vi "Set Level.vi"(6 "Output Channel":T1, 8 "error in (no error)":errorcluster, 9 "Slew (V/s)":dbl, 10 "Level (V)":dbl, 11 "RP100 in":refnum<class "RP100.lvclass">) -> (0 "error out":errorcluster, 3 "RP100 out":refnum<class "RP100.lvclass">)   [LabVIEW 2019, in "RP100.lvclass"]
doc: "Set the output <b>Level</b> with <b>Slew</b> rate on the selected <b>Output Channel</b>"
uses:
  RP100.lvclass
  C:/Program Files (x86)/National Instruments/LabVIEW 2019/user.lib/LevyLab/Levylab Instruments/SMOs/Instrument/Instrument.lvclass
  Typedefs/Output Channel--Enum.ctl
  Typedefs/Commands--Enum.ctl
  Typedefs/setLevel--Cluster.ctl
  <userlib>/LevyLab/Instrument Framework/SMOs/Instrument/Instrument.lvclass/Instrument.ctl
  561c9bc1-5633-4095-b2f1-945bf898e835.vi
  561c9bc1-5633-4095-b2f1-945bf898e835.vi/237b59a2-2d82-4dc4-8148-7fb860610e54.vi
  561c9bc1-5633-4095-b2f1-945bf898e835.vi/237b59a2-2d82-4dc4-8148-7fb860610e54.vi/3b1c6db6-cacd-475f-9763-016a014ff714.vi
  <userlib>/LevyLab/Instrument Framework/SMOs/Instrument/API/Send and Receive.vi
  561c9bc1-5633-4095-b2f1-945bf898e835.vi/237b59a2-2d82-4dc4-8148-7fb860610e54.vi/3b1c6db6-cacd-475f-9763-016a014ff714.vi/893b43f6-e8c9-4ae5-9cfa-c1df81c9f79f.vi
  561c9bc1-5633-4095-b2f1-945bf898e835.vi/237b59a2-2d82-4dc4-8148-7fb860610e54.vi/3b1c6db6-cacd-475f-9763-016a014ff714.vi/1a03cde0-227b-4f55-9e3b-b0f9a698a2d0.vi
  <userlib>/LevyLab/Instrument Framework/SMOs/Instrument/API/Enum to String.vi
  <userlib>/LevyLab/Instrument Framework/SMOs/RemoteControl/API/Send and Receive.vi
  <vilib>/Utility/Data Type/Get Type Information.vi
  <vilib>/JDP Science/JSONtext/JSON text to Variant.vi
  <vilib>/JDP Science/JSONtext/LVClass Serializer/JSONtext LVClass Serializer.lvclass
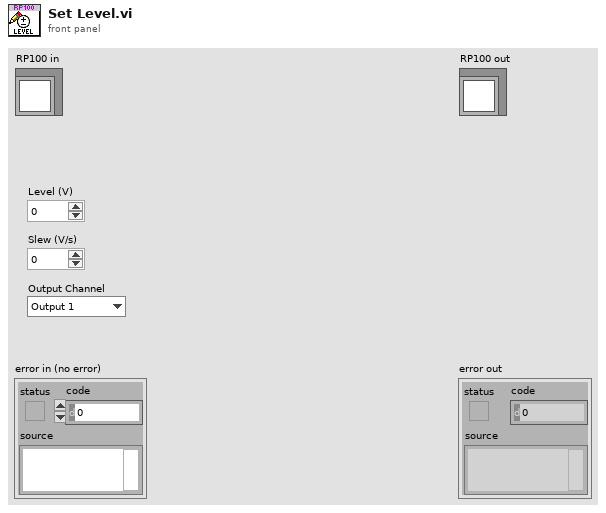
[diagram p1: front panel]
types:
  T1 = typedef "RP100.lvclass/Output Channel--Enum.ctl" = enum16{"Output 1", "Output 2"}
  T2 = typedef "RP100.lvclass/setLevel--Cluster.ctl" = cluster{"Output Channel":T1, "Level (V)":dbl, "Slew (V/s)":dbl}
  T3 = typedef "RP100.lvclass/Commands--Enum.ctl" = enum16{"setStrain", "getStrain", "setLevel", "getLevel"}
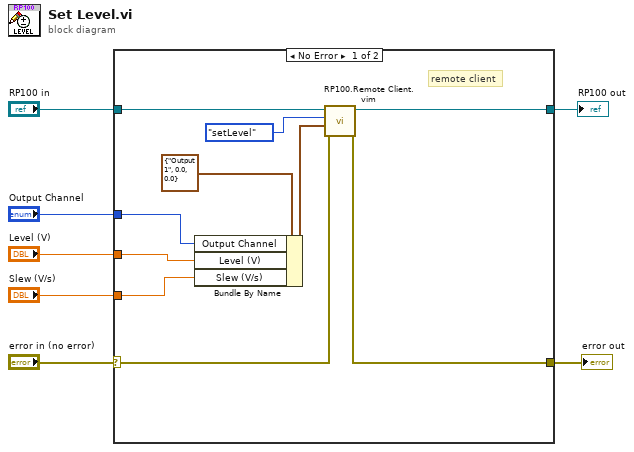
[diagram p0: block diagram]
diagram:
  n1 = case shown="No Error" "error in (no error)" {
    selector: "error in (no error)" -> [w15 w19]
    tunnel: [w14 w19] -> w6
    tunnel: "Level (V)" -> [w9 _]
    tunnel: "RP100 in" -> [w17 w18]
    tunnel: [w16 w18] -> w3
    tunnel: "Slew (V/s)" -> [w8 _]
    tunnel: "Output Channel" -> [w10 _]
    frame No Error {
      # "remote client"
      n2 = Bundle By Name(cluster=T2 {"Output Channel"=enum."Output 1", "Level (V)"=0.0, "Slew (V/s)"=0.0} ("setLevel"), "Output Channel"=w10, "Level (V)"=w9, "Slew (V/s)"=w8) -> (w11:T2)
      n3 = call "RP100.Remote Client.vim"("error in (no error)"=w15, "params"=w11, "Commands"=Commands--Enum."setLevel", "RP100 in"=w17) -> ("error out"=w14:errorcluster, "RP100 out"=w16:refnum<class "RP100.lvclass">)  [unwired: 5 in, 1 out]
    }
    frame Error {
    }
  }
  "error out" <- w6
  "RP100 out" <- w3
